vi "Save Results to TDMS.vi"(1 "measurement configuration":T2={"DUT setup time"=1.0, "Nominal output voltage"=3.3, "Source pin name"="", "Source current limit"=0.25, "Source maximum power"=300.0, "Source sample rate"=1800000.0, "Source voltage set point 1"=7.0, "Source voltage set point 2"=20.0, "Source voltatge pulse duration"=0.005, "Source voltage delay t1"=0.005, "Source voltage delay t2"=0.005, "Source voltage falling slew rate"=50000.0, "Source voltage rising slew rate"=50000.0, "Source transient response"=1042, "Source voltage gain bandwidth"=2000.0, "Source voltage compensation frequency"=3530.0, "Source voltage pole-zero ratio"=2.0, "Load pin name"="", "Load voltage limit range"=4.0, "Load current level range"=4.0, "Load current level"=0.03, "Load transient response"=1042, "Load current gain bandwidth"=14000.0, "Load current compensation frequency"=180000.0, "Load current pole-zero ratio"=0.3, "Pin Names for Scope"=[], "vertical range"=[], "vertical offset"=[], "probe attenuation"=[], "vertical coupling"=[], "channel enabled"=[], "input impedance"=[], "max input frequency"=[], "min sample rate"=[], "reference position"=[], "min record length"=[], "enforce realtime"=[]} {"input impedance" items=["1 mega ohm"=0, "50 ohms"=2]; "vertical coupling" items=["AC", "DC", "Ground"]; "Source voltage delay t1" format="%#_8g"; "Load transient response" items=["Slow"=1041, "Normal"=1038, "Fast"=1039, "Custom"=1042]; "Source transient response" items=["Slow"=1041, "Normal"=1038, "Fast"=1039, "Custom"=1042]}, 3 "measurement results":T1={"dt"=0.0, "Load voltages"=[], "Undershoot load voltage"=0.0, "Overshoot load voltage"=0.0, "Source voltages"=[0.0], "waveform pins"=[], "waveform sites"=[], "waveform t0 array"=[], "waveform dt array"=[], "waveform length array"=[], "concatenated waveform Y"=[]}, 4 "Scope waveforms":waveform(dbl)[](array[waveform]), 5 "error in (no error)":errorcluster) -> (19 "error out":errorcluster)   [LabVIEW 2021, in "Line Transient Response with Pin Map.lvlib"]
uses:
  Line Transient Response with Pin Map.lvlib
  Measurement Configuration.ctl
  <instrlib>/niScope/Controls/niScope vertical coupling.ctl
  Measurement Results.ctl
  <vilib>/Utility/sysdir.llb/System Directory Type.ctl
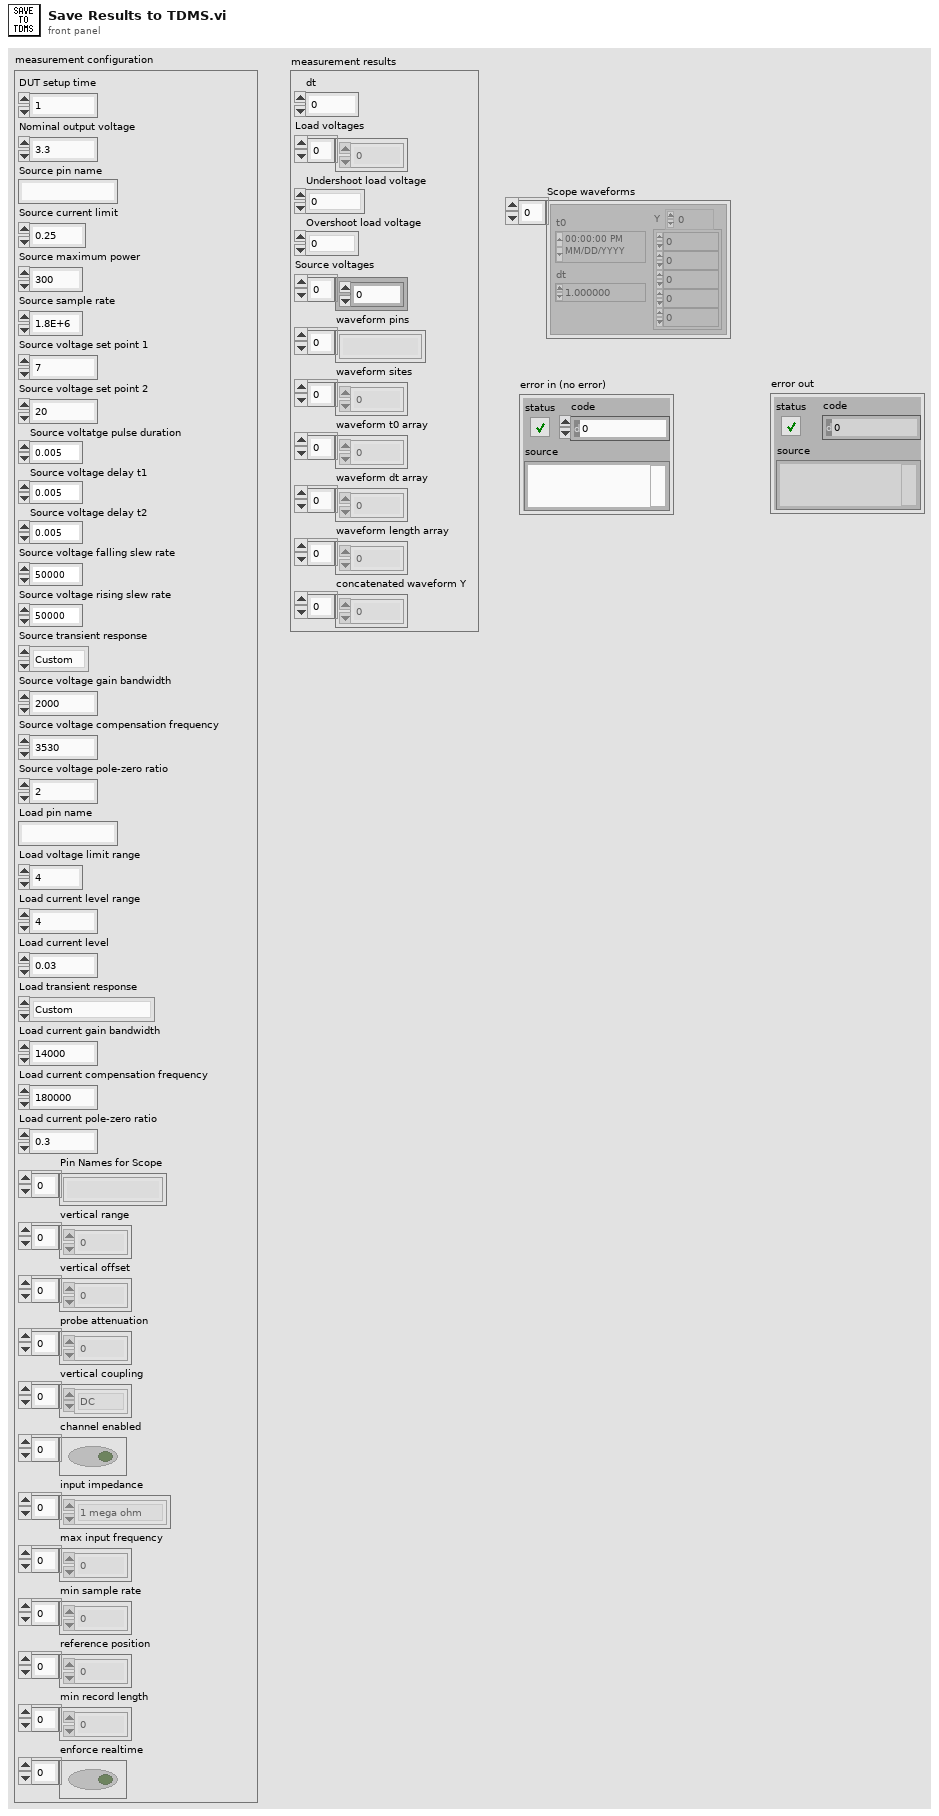
[diagram p1: front panel]
types:
  T1 = typedef "Line Transient Response with Pin Map.lvlib/Measurement Results.ctl" = cluster{"dt":dbl, "Load voltages":dbl[], "Undershoot load voltage":dbl, "Overshoot load voltage":dbl, "Source voltages":dbl[], "waveform pins":string[], "waveform sites":i32[], "waveform t0 array":dbl[], "waveform dt array":dbl[], "waveform length array":i32[], "concatenated waveform Y":dbl[]}
  T2 = typedef "Line Transient Response with Pin Map.lvlib/Measurement Configuration.ctl" = cluster{"DUT setup time":dbl, "Nominal output voltage":dbl, "Source pin name":string, "Source current limit":dbl, "Source maximum power":dbl, "Source sample rate":dbl, "Source voltage set point 1":dbl, "Source voltage set point 2":dbl, "Source voltatge pulse duration":dbl, "Source voltage delay t1":dbl, "Source voltage delay t2":dbl, "Source voltage falling slew rate":dbl, "Source voltage rising slew rate":dbl, "Source transient response":i32, "Source voltage gain bandwidth":dbl, "Source voltage compensation frequency":dbl, "Source voltage pole-zero ratio":dbl, "Load pin name":string, "Load voltage limit range":dbl, "Load current level range":dbl, "Load current level":dbl, "Load transient response":i32, "Load current gain bandwidth":dbl, "Load current compensation frequency":dbl, "Load current pole-zero ratio":dbl, "Pin Names for Scope":string[], "vertical range":dbl[], "vertical offset":dbl[], "probe attenuation":dbl[], "vertical coupling":T3[], "channel enabled":bool[], "input impedance":u32[], "max input frequency":dbl[], "min sample rate":dbl[], "reference position":dbl[], "min record length":i32[], "enforce realtime":bool[]}
  T3 = typedef "niScope vertical coupling.ctl" = i32
  T4 = typedef "System Directory Type.ctl" = i32
  T5 = enum16{"open", "open or create", "create or replace", "create", "open (read-only)"}
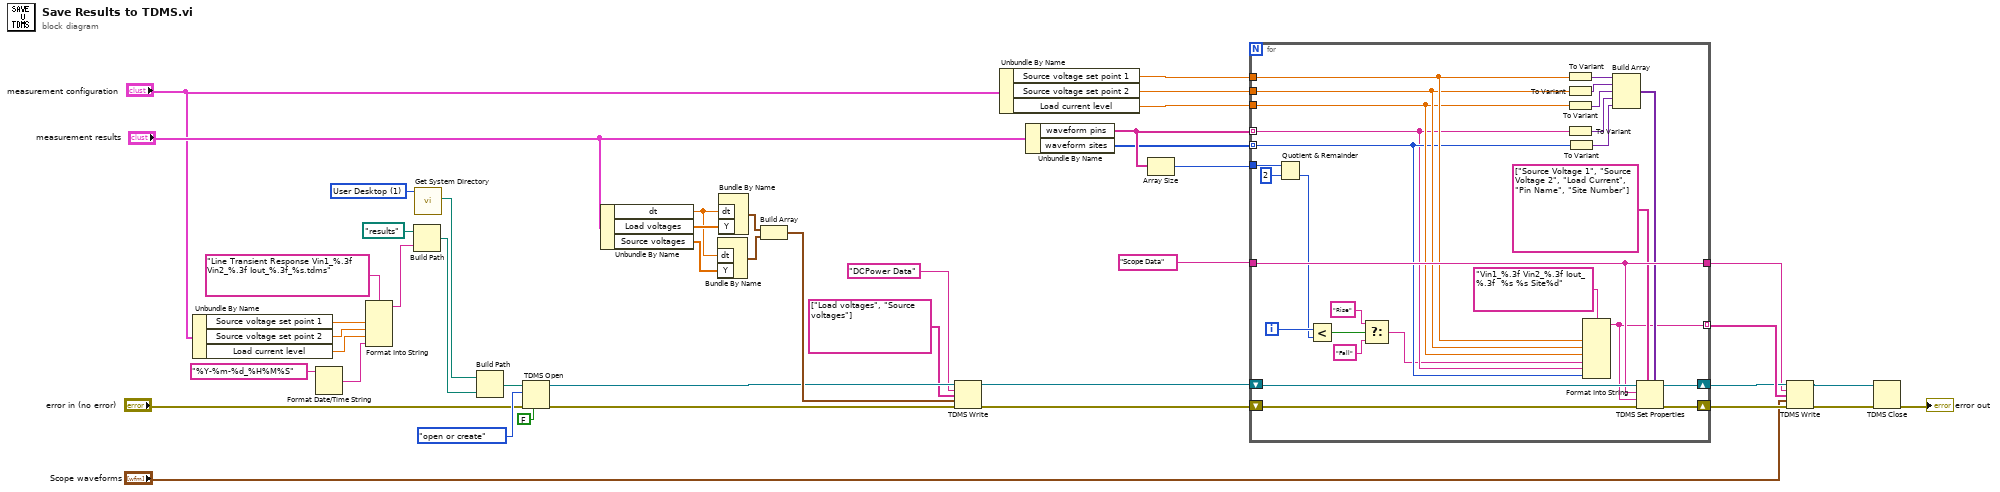
[diagram p0: block diagram]
diagram:
  w24 = T4 1 items=["User Home"=0, "User Desktop"=1, "User Documents"=2, "User Application Data"=3, "User Preferences"=4, "User Temporary"=5, "Public Documents"=6, "Public Application Data"=7, "Public Preferences"=8, "Public Cache"=13, "System Core Libraries"=9, "System Installed Libraries"=10, "Application Files"=11, "Boot Volume Root"=12] ("system directory type")
  n1 = Unbundle By Name("measurement configuration") -> ("Source voltage set point 1"=w34:dbl, "Source voltage set point 2"=w33:dbl, "Load current level"=w32:dbl)
  n2 = Format Date/Time String(time format string (%c)="%Y-%m-%d_%H%M%S") -> (date/time string=w1:string)  [unwired: 2 in]
  n3 = Format Into String(format string="Line Transient Response Vin1_%.3f Vin2_%.3f Iout_%.3f_%s.tdms", w34, w33, w32, w1) -> (resulting string=w30:string)  [unwired: 2 in, 1 out]
  n4 = Build Path(base path=path "results", name or relative path=w30) -> (appended path=w29:path)
  n5 = call <vilib>:"Get System Directory.vi"("system directory type"=w24) -> ("system directory"=w23:path)  [unwired: 10 in]
  n6 = Build Path(base path=w23, name or relative path=w29) -> (appended path=w42:path)
  n7 = TDMS Open(6:FALSE ("disable buffering? (T)"), 8:"error in (no error)", 10:T5."open or create" ("operation (0:open)"), 11:w42) -> (0:w27:errorcluster, 3:w28:refnum<k34>)  [unwired: 3 in]
  n8 = Unbundle By Name("measurement results") -> ("dt"=w39:dbl, "Load voltages"=w41:dbl[], "Source voltages"=w40:dbl[])
  n9 = Bundle By Name("dt"=w39, "Y"=w40) -> (w37:waveform(dbl))  [unwired: 1 in]
  n10 = Bundle By Name("dt"=w39, "Y"=w41) -> (w38:waveform(dbl))  [unwired: 1 in]
  n11 = Build Array(w38, w37) -> (w36:waveform(dbl)[])
  n12 = TDMS Write(0:w28, 5:"DCPower Data" ("group name in (Untitled)"), 7:string[] ["Load voltages", "Source voltages"], 9:w36, 11:w27) -> (4:w12:refnum<k34>, 15:w11:errorcluster)  [unwired: 1 in, 2 out]
  n13 = Unbundle By Name("measurement configuration") -> ("Source voltage set point 1"=w8:dbl, "Source voltage set point 2"=w7:dbl, "Load current level"=w6:dbl)
  n14 = Unbundle By Name("measurement results") -> ("waveform pins"=w5:string[], "waveform sites"=w4:i32[])
  n15 = Array Size(array=w5) -> (size(s)=w3:i32)
  n16 = for {
    tunnel: w8 -> [w64]
    tunnel: w7 -> [w63]
    tunnel: w5 -> [w53] mode=indexing
    tunnel: [w59] -> w22 mode=indexing
    shift-right: [w69] -> w21
    shift-left: w12 -> [w70]
    shift-right: [w67] -> w20
    shift-left: w11 -> [w68]
    tunnel: "Scope Data" ("group name in (Untitled)") -> [w66]
    tunnel: [w66] -> w19
    tunnel: w4 -> [w54] mode=indexing
    tunnel: w6 -> [w55]
    tunnel: w3 -> [w52]
    i -> [w50]
    n17 = Quotient & Remainder(x=w52, y=2) -> (floor(x/y)=w49:i32)  [unwired: 1 out]
    n18 = Less?(x=w50, y=w49) -> (x < y?=w46:bool)
    n19 = Select(t="Rise", s=w46, f="Fall") -> (s? t:f=w45:string)
    n20 = To Variant(anything=w64) -> (Variant=w62:variant)
    n21 = To Variant(anything=w63) -> (Variant=w61:variant)
    n22 = To Variant(anything=w55) -> (Variant=w56:variant)
    n23 = To Variant(anything=w53) -> (Variant=w58:variant)
    n24 = To Variant(anything=w54) -> (Variant=w57:variant)
    n25 = Format Into String(format string="Vin1_%.3f Vin2_%.3f Iout_%.3f  %s %s Site%d", w64, w63, w55, w45, w53, w54) -> (resulting string=w59:string)  [unwired: 2 in, 1 out]
    n26 = Build Array(w62, w61, w56, w58, w57) -> (w60:variant[])
    n27 = TDMS Set Properties(5:w60, 7:string[] ["Source Voltage 1", "Source Voltage 2", "Load Current", "Pin Name", "Site Number"] ("property names"), 8:w68, 9:w59, 10:w66, 11:w70) -> (0:w67:errorcluster, 3:w69:refnum<k34>)  [unwired: 2 out]
  }
  n28 = TDMS Write(0:w21, 5:w19, 7:w22, 9:"Scope waveforms", 11:w20) -> (4:w15:refnum<k34>, 15:w14:errorcluster)  [unwired: 1 in, 2 out]
  n29 = TDMS Close(8:w14, 11:w15) -> (0:→"error out":errorcluster)  [unwired: 1 out]
